vi "WriteButtonBar.vi"(8 "ErrorIn":errorcluster, 10 "ButtonBar":refnum<class "ButtonCollection.lvclass"> caption="Object Out", 11 "ReferenceIn":refnum<class "VerticalButtonBar.lvclass">) -> (0 "ErrorOut":errorcluster, 3 "ReferenceIn":refnum<class "VerticalButtonBar.lvclass">)   [LabVIEW 2021, in "VerticalButtonBar.lvclass"]
uses:
  VerticalButtonBar.lvclass
  ButtonCollection/ButtonCollection.lvclass
  VerticalButtonBar.lvclass/VerticalButtonBar.ctl
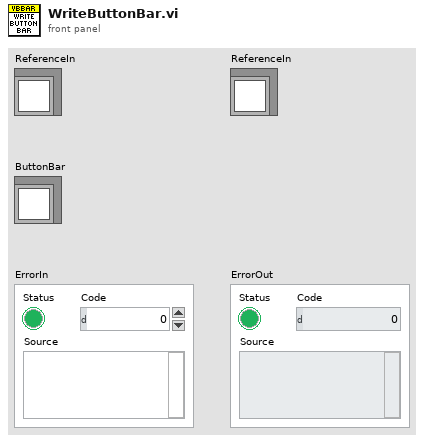
[diagram p1: front panel]
types:
  T1 = typedef "VerticalButtonBar.lvclass/ObjectAttributes.ctl" = cluster{"Interfaces":cluster{"IDockGUI":refnum<class "IDockGUI.lvclass">, "Authorizer":refnum<class "IAuthorization.lvclass">}, "Locals":cluster{"ButtonBar":refnum<class "ButtonCollection.lvclass">, "BaseConfigurationPath":path, "Labels":cluster{"Label":string, "Value":string}[]}, "Persistent":cluster{"ButtonDefinitionFile":string}}
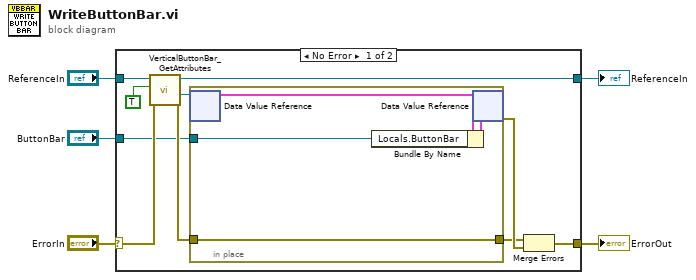
[diagram p0: block diagram]
diagram:
  n1 = case shown="No Error" "ErrorIn" {
    selector: "ErrorIn" -> [w15 w21]
    tunnel: [w13 w21] -> w4
    tunnel: [w9 w20] -> w2
    tunnel: "ReferenceIn" -> [w10 w20]
    tunnel: "ButtonBar" -> [w6 _]
    frame No Error {
      n2 = call "VerticalButtonBar_GetAttributes.vi"("ErrorIn"=w15, "OnlyGetDvrReference(False)"=TRUE, "ReferenceIn"=w10) -> ("ErrorOut"=w12:errorcluster, "DataRef"=w7:refnum<data-value>, "ReferenceOut"=w9:refnum<class "VerticalButtonBar.lvclass">)  [unwired: 5 in, 1 out]
      n3 = in-place {
        in-place-border: w6 -> [w16]
        in-place-border: w12 -> [w19]
        in-place-border: [w19] -> w11
        n4 = in-place-dvr #1(w7) -> (w17:T1)  [unwired: 1 out]
        n5 = Bundle By Name(cluster=w17, "Locals.ButtonBar"=w16) -> (w18:T1)
        n6 = in-place-dvr #1(w18) -> (w14:errorcluster)  [unwired: 1 out]
      }
      n7 = Merge Errors(w11, w14) -> (w13:errorcluster)
    }
    frame Error {
    }
  }
  "ErrorOut" <- w4
  "ReferenceIn" <- w2
